vi "Demo.vi"() -> ()   [LabVIEW 2020]
panel:
  out "Output Image File":path
  out "Base64String From File":string
  in  "Input Image File":path=path "demo.png"
  out "DecodedImage":picture
  out "Base64String":string
  out "InputImage":picture
  # "Base64 Image Data Conversion  (LVImage)"
  # "Encode"
  # "Decode"
  # "Base64 Image Data Conversion  (From/To File)"
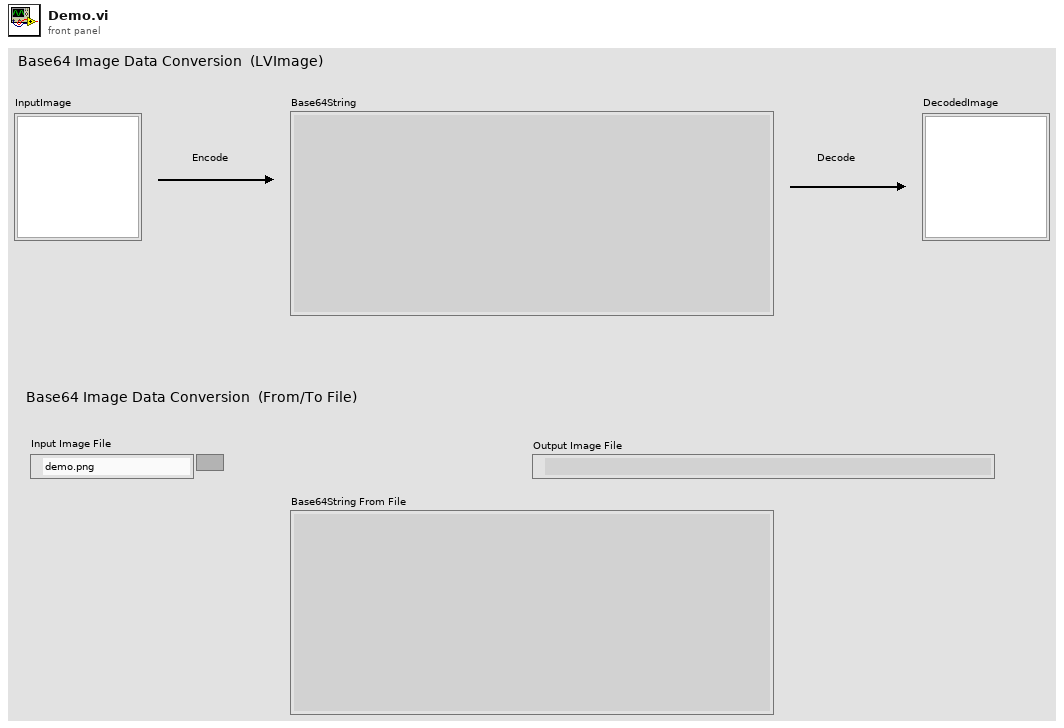
[diagram p1: front panel]
types:
  T1 = typedef "imagedata.ctl" = cluster{"image type":i32, "image depth":i32, "image":u8[], "mask":u8[], "colors":u32[], "Rectangle":cluster{"left":i16, "top":i16, "right":i16, "bottom":i16}}
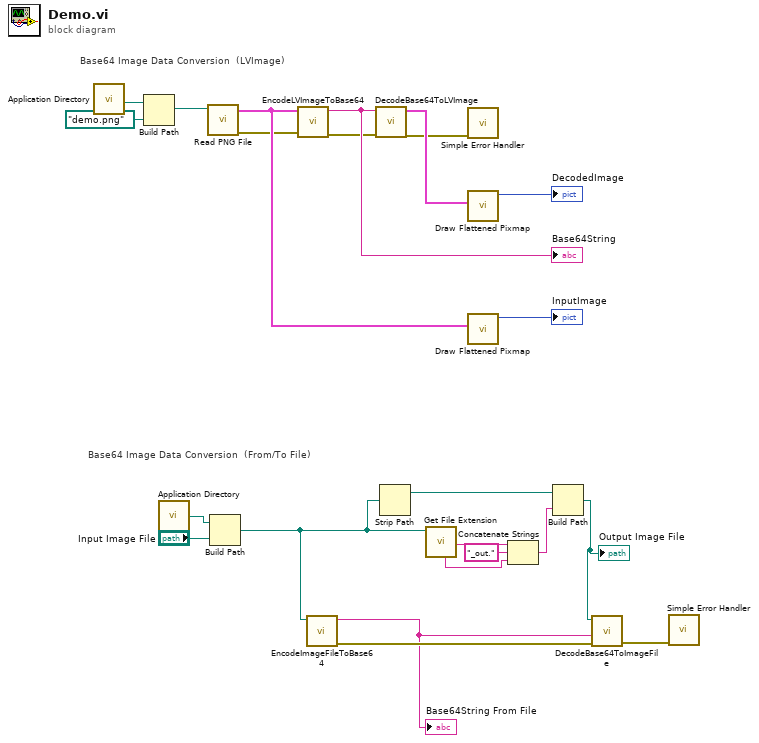
[diagram p0: block diagram]
diagram:
  # "Base64 Image Data Conversion  (From/To File)"
  # "Base64 Image Data Conversion  (LVImage)"
  n1 = call <vilib>:"Application Directory.vi"() -> ("Application Directory"=w23:path)
  n2 = Build Path(base path=w23, name or relative path=path "demo.png") -> (appended path=w21:path)
  n3 = call <vilib>:"Application Directory.vi"() -> ("Application Directory"=w12:path)
  n4 = call <vilib>:"Read PNG File.vi"("path to PNG file"=w21) -> ("error out"=w15:errorcluster, "image data"=w19:T1)  [unwired: 8 in, 1 out]
  n5 = Build Path(base path=w12, name or relative path="Input Image File") -> (appended path=w7:path)
  n6 = call "EncodeLVImageToBase64.vi"("error in (no error)"=w15, "LVImage"=w19) -> ("error out"=w14:errorcluster, "Base64String"=w18:string)  [unwired: 8 in]
  "Base64String" <- w18
  n7 = call "EncodeImageFileToBase64.vi"("ImagePath"=w7) -> ("error out"=w4:errorcluster, "Base64String"=w3:string)  [unwired: 9 in]
  "Base64String From File" <- w3
  n8 = call "DecodeBase64ToLVImage.vi"("error in (no error)"=w14, "Base64String"=w18) -> ("error out"=w13:errorcluster, "LVImage"=w16:T1)  [unwired: 8 in]
  n9 = Strip Path(path=w7) -> (stripped path=w6:path)  [unwired: 1 out]
  n10 = call <vilib>:"Get File Extension.vi"("file"=w7) -> ("filename without extension"=w10:string, "unmodified file extension"=w8:string)  [unwired: 6 in, 3 out]
  n11 = call <vilib>:"Simple Error Handler.vi"("error in (no error)"=w13) -> ()  [unwired: 4 in, 5 out]
  n12 = call <vilib>:"Draw Flattened Pixmap.vi"("image data"=w16) -> ("new picture"=→"DecodedImage":picture)  [unwired: 8 in]
  n13 = call <vilib>:"Draw Flattened Pixmap.vi"("image data"=w19) -> ("new picture"=→"InputImage":picture)  [unwired: 8 in]
  n14 = Concatenate Strings(w10, "_out." ("string"), w8) -> (w5:string)
  n15 = Build Path(base path=w6, name or relative path=w5) -> (appended path=w2:path)
  "Output Image File" <- w2
  n16 = call "DecodeBase64ToImageFile.vi"("error in (no error)"=w4, "Base64String"=w3, "Output FilePath"=w2) -> ("error out"=w1:errorcluster)  [unwired: 7 in, 1 out]
  n17 = call <vilib>:"Simple Error Handler.vi"("error in (no error)"=w1) -> ()  [unwired: 4 in, 5 out]
